vi "PmacCommSendStr.vi"(1 "Command String":string, 2 "Device Number i32 (0)":i32 min=0) -> (0 "Device Number i32 (0)":i32 min=0)   [LabVIEW 2020]
doc: "Send Command String to PMAC. If Command String is the empty string nothing is sent. The output Device Number is a copy of input Device Number to allow sequencing of commands to PMAC."
uses:
  Builds/5-8-13/data/PComm32W.dll
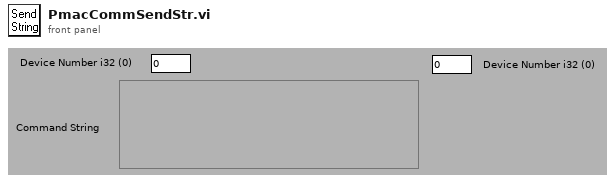
[diagram p1: front panel]
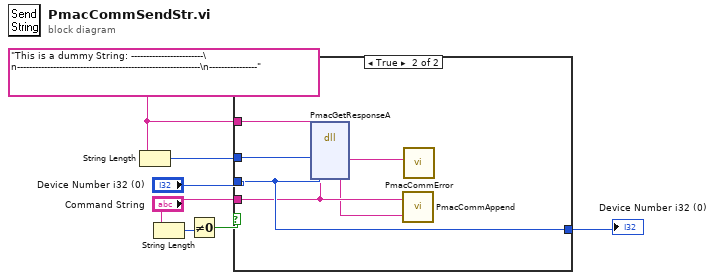
[diagram p0: block diagram]
diagram:
  w3 = "This is a dummy String: ------------------------\n-------------------------------------------------------------\n----------------"
  n1 = String Length(string=w3) -> (length=w2:i32)
  n2 = String Length(string="Command String") -> (length=w4:i32)
  n3 = Not Equal To 0?(x=w4) -> (x != 0?=w7:bool)
  n4 = case shown="True" w7 {
    tunnel: "Device Number i32 (0)" -> [w8 w12]
    tunnel: "Command String" -> [_ w10]
    tunnel: w2 -> [_ w13]
    tunnel: w3 -> [_ w11]
    tunnel: [w8 w12] -> w1
    frame False {
    }
    frame True {
      n5 = dll-call lib="C:/NUWAR_Master/Builds/5-8-13/data/PComm32W.dll" fn="PmacGetResponseA"("DeviceNumber"=w12, "CommandString"=w11, "MaxStringLength"=w13, "ResponseString"=w10) -> ("CommandString"=w9:string)  [unwired: 5 in, 4 out]
      n6 = call "PmacCommAppend.vi"("Response String"=w9, "Command String"=w10) -> ()
      n7 = call "PmacCommError.vi"("Input String"=w9) -> ()  [unwired: 4 out]
    }
  }
  "Device Number i32 (0)" <- w1
